vi "Polygon Intersection_Incr Index.vi"(9 "polygon size":i32, 10 "incr":i32, 11 "index":i32) -> (3 "incr index":i32)   [LabVIEW 2017, in "NI_AAL_Geometry.lvlib"]
uses:
  <vilib>/Analysis/NI_AAL_Geometry.lvlib
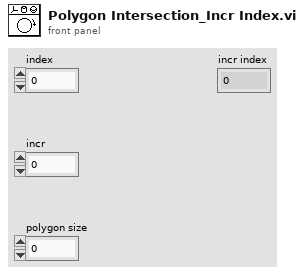
[diagram p1: front panel]
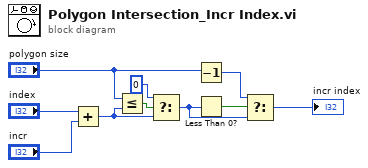
[diagram p0: block diagram]
diagram:
  n1 = Add(x="index", y="incr") -> (x+y=w7:i32)
  n2 = Less Or Equal?(x="polygon size", y=w7) -> (x <= y?=w10:bool)
  n3 = Select(t=0, s=w10, f=w7) -> (s? t:f=w4:i32)
  n4 = Decrement(x="polygon size") -> (x-1=w3:i32)
  n5 = Less Than 0?(x=w4) -> (x < 0?=w5:bool)
  n6 = Select(t=w3, s=w5, f=w4) -> (s? t:f=→"incr index":i32)
